vi "Sine wave sub vi.vi"(11 "Numeric":dbl) -> ()   [LabVIEW 2018]
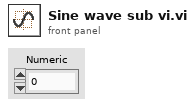
[diagram p1: front panel]
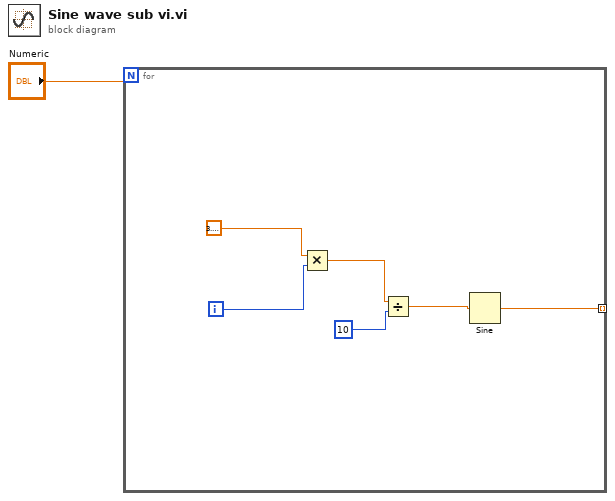
[diagram p0: block diagram]
diagram:
  n1 = for {
    N: "Numeric" -> [_]
    tunnel: [w2] -> _ mode=indexing
    i -> [w7]
    n2 = Multiply(x=3.141592653589793, y=w7) -> (x*y=w5:dbl)
    n3 = Divide(x=w5, y=10) -> (x/y=w3:dbl)
    n4 = Sine(x=w3) -> (sin(x)=w2:dbl)
  }
